vi "Test  PCAN Read RAW Frame.vi"(11 "Test Case In":refnum<class "Test PCAN.lvclass">) -> (0 "error out":errorcluster, 3 "Test Case Out":refnum<class "Test PCAN.lvclass">)   [LabVIEW 2025, in "Test PCAN.lvclass"]
uses:
  Test PCAN.lvclass
  C:/Program Files/National Instruments/LabVIEW 2025/vi.lib/Astemes/LUnit/Test Case.lvclass
  Source/Communicator/Communicator.lvclass
  Source/Configure Strategies/PCAN-USB Read-Write Raw CAN Frame Strategy/PCAN-USB Read-Write Raw CAN Frame Strategy.lvclass
  D:/git/HAL/Source/Interfaces/IConfigure/IConfigure.lvclass
  <vilib>/Astemes/LUnit/Test Case.lvclass/Test Case.ctl
  <vilib>/Astemes/LUnit/Append Pass Result.vi
  <vilib>/Astemes/LUnit/Append Fail Result.vi
  <vilib>/Astemes/LUnit/Run In UI.vi
  <vilib>/Utility/error.llb/Clear Errors.vi
  Source/Interfaces/IMessage/IMessage.lvclass
  <vilib>/Astemes/LUnit/Test Case.lvclass
panel:
  out "Identifier":string
  out "Data":u8[](array[numeric]) format="%.0x"
  out "Timestamp":timestamp
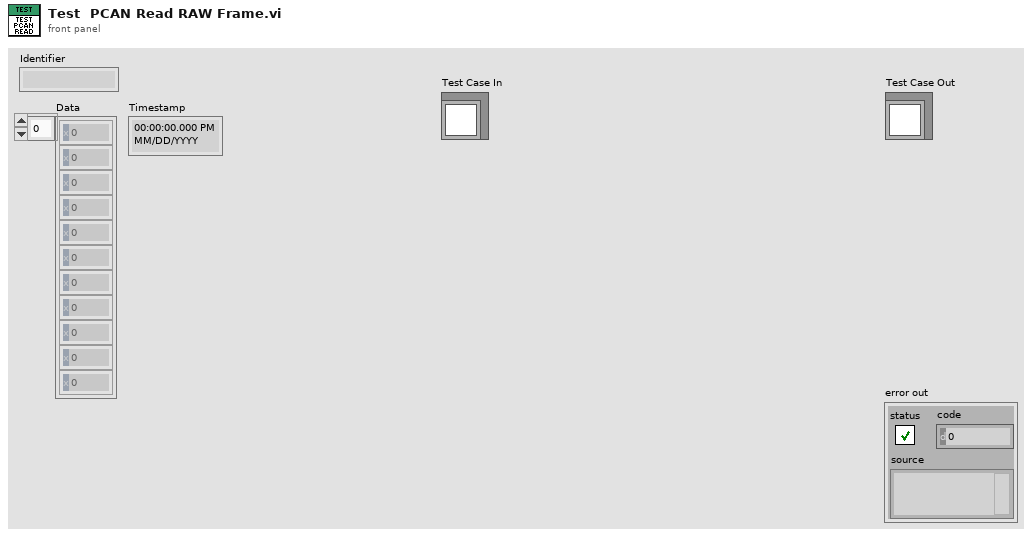
[diagram p1: front panel]
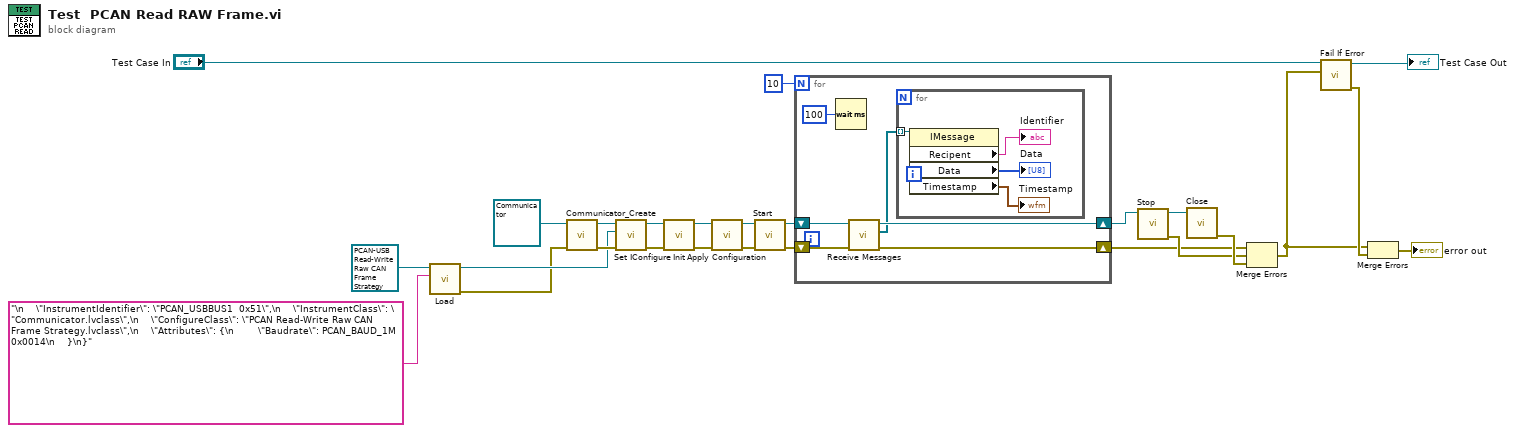
[diagram p0: block diagram]
diagram:
  n1 = call-dynamic "Load.vi"("Source"="\n    \"InstrumentIdentifier\": \"PCAN_USBBUS1  0x51\",\n    \"InstrumentClass\": \"Communicator.lvclass\",\n    \"ConfigureClass\": \"PCAN Read-Write Raw CAN Frame Strategy.lvclass\",\n    \"Attributes\": {\n        \"Baudrate\": PCAN_BAUD_1M 0x0014\n    }\n}", "PCAN-USB Read-Write Raw CAN Frame Strategy in"=refnum<class "PCAN-USB Read-Write Raw CAN Frame Strategy.lvclass"> refnum ("PCAN-USB Read-Write Raw CAN Frame Strategy")) -> ("error out"=w8:errorcluster, "PCAN-USB Read-Write Raw CAN Frame Strategy out"=w25:refnum<class "PCAN-USB Read-Write Raw CAN Frame Strategy.lvclass">)  [unwired: 8 in]
  n2 = call "Communicator_Create.vi"("Error In"=w8, "Communicator in"=refnum<class "Communicator.lvclass"> refnum ("PCAN-USB")) -> ("Error Out"=w26:errorcluster, "Communicator out"=w16:refnum<class "Communicator.lvclass">)  [unwired: 8 in]
  n3 = call-dynamic "Set IConfigure.vi"("Error In"=w26, "IConfigure"=w25, "Communicator in"=w16) -> ("Error Out"=w24:errorcluster, "Communicator out"=w23:refnum<class "Communicator.lvclass">)  [unwired: 7 in]
  n4 = call-dynamic "Init.vi"("Error In"=w24, "Communicator in"=w23) -> ("Error Out"=w22:errorcluster, "Communicator out"=w21:refnum<class "Communicator.lvclass">)  [unwired: 8 in]
  n5 = call-dynamic "Apply Configuration.vi"("Error In"=w22, "Communicator in"=w21) -> ("Error Out"=w13:errorcluster, "Communicator out"=w14:refnum<class "Communicator.lvclass">)  [unwired: 8 in]
  n6 = call-dynamic "Start.vi"("Error In"=w13, "Communicator in"=w14) -> ("Error Out"=w18:errorcluster, "Communicator out"=w19:refnum<class "Communicator.lvclass">)  [unwired: 8 in]
  n7 = for {
    N: 10 -> [_]
    shift-right: [w30] -> w17
    shift-left: w19 -> [w32]
    shift-right: [w29] -> w10
    shift-left: w18 -> [w31]
    n8 = Wait (ms)(milliseconds to wait=u32 100) -> ()  [unwired: 1 out]
    n9 = call-dynamic "Receive Messages.vi"("Error In"=w31, "Communicator in"=w32) -> ("Error Out"=w29:errorcluster, "Messages"=w28:refnum<class "IMessage.lvclass">[], "Communicator out"=w30:refnum<class "Communicator.lvclass">)  [unwired: 7 in]
    n10 = for {
      tunnel: w28 -> [w36] mode=indexing
      n11 = property class="IMessage"(reference=w36) -> ("Recipent"=→"Identifier":string, "Data"=→"Data":u8[], "Timestamp"=→"Timestamp":timestamp)  [unwired: 1 in, 2 out]
    }
  }
  n12 = call-dynamic "Stop.vi"("Communicator in"=w17) -> ("Error Out"=w11:errorcluster, "Communicator out"=w15:refnum<class "Communicator.lvclass">)  [unwired: 9 in]
  n13 = call-dynamic "Close.vi"("Communicator in"=w15) -> ("Error Out"=w12:errorcluster)  [unwired: 9 in, 1 out]
  n14 = Merge Errors(w10, w11, w12) -> (w3:errorcluster)
  n15 = call <vilib>:"Fail If Error.vi"("Assert error"=w3, "LUnit Test Case In"="Test Case In") -> ("error out"=w5:errorcluster, "LUnit Test Case Out"=→"Test Case Out":refnum<class "Test PCAN.lvclass">)  [unwired: 8 in]
  n16 = Merge Errors(w3, w5) -> (→"error out":errorcluster)
